vi "Finish.vi"   [LabVIEW 2014]
doc: "This VI is called just before exiting. It is expected to close I/O refnum, save collected data, etc."
uses:
  <vilib>/Rock Robotics/WPI/Joystick/WPI_JoystickGetSetRefNum.vi
  <vilib>/Rock Robotics/WPI/RobotDrive/WPI_RobotDriveGetSetRefNum.vi
  <vilib>/Rock Robotics/WPI/Compressor/WPI_CompressorGetSetRefNum.vi
types:
  T1 = typedef "WPI_JoystickDevRef.ctl" = cluster{"Device":T2}
  T2 = typedef "WPI_JoystickDeviceEnum.ctl" = enum16{"USB 0", "USB 1", "USB 2", "USB 3", "USB 4", "USB 5"}
  T3 = typedef "WPI_RobotDriveDevRef.ctl" = cluster{"DevStatus":errorcluster, "Motors[]":T4[], "Square Inputs":bool, "Max Output":dbl}
  T4 = typedef "WPI_MotorControlDeviceRef.ctl" = cluster{"DeviceStatus":errorcluster, "Type":T5, "PWM":cluster{"Controller":T6, "PWM Channel":T7, "DeadBand":T8}, "CAN":cluster{"Device Number":u8, "Control Mode":T9, "Semaphore":T10, "Max Vout":dbl, "TalonSRX Control Mode":T11}, "Invert":bool, "TransformRef":T12, "InvTransformRef":T12}
  T5 = typedef "WPI_MotorControlType.ctl" = enum16{"PWM", "CAN", "CANTalonSRX"}
  T6 = typedef "FPGA_TypedefDigitalModule.ctl" = enum16{"Controller 1"}
  T7 = typedef "FPGA_DIOPWMChannel.ctl" = enum8{"PWM 0", "PWM 1", "PWM 2", "PWM 3", "PWM 4", "PWM 5", "PWM 6", "PWM 7", "PWM 8", "PWM 9", "PWM MXP 0", "PWM MXP 1", "PWM MXP 2", "PWM MXP 3", "PWM MXP 4", "PWM MXP 5", "PWM MXP 6", "PWM MXP 7", "PWM MXP 8", "PWM MXP 9", "Invalid"}
  T8 = typedef "WPI_PWMDeadband.ctl" = cluster{"Name":string, "maxPositivePwm":i32, "minPositivePwm":i32, "centerPwm":i32, "maxNegativePwm":i32, "minNegativePwm":i32, "angularRange":u16}
  T9 = typedef "WPI_CANJaguar_ControlMode.ctl" = enum8{"Percent VBus", "Current", "Speed", "Position", "Voltage"}
  T10 = typedef "Semaphore RefNum" = refnum<k1>
  T11 = typedef "WPI_CANTalonSRX_APIControlMode.ctl" = enum8{"Percent VBus", "Speed", "Position", "Slave", "Unchanged / Invalid"}
  T12 = typedef "WPI_PWMTransform_ConPane.ctl" = refnum<vi>
  T13 = typedef "WPI_ServoDeviceRef.ctl" = cluster{"DeviceStatus":errorcluster, "Controller":T6, "PWM Channel":T7, "DeadBand":T8}
  T14 = typedef "WPI_DigitalInputDevRef.ctl" = cluster{"DevStatus":errorcluster, "DIO Channel":T15, "Controller":T6}
  T15 = typedef "FPGA_DIOChannel.ctl" = enum8{"DIO 0", "DIO 1", "DIO 2", "DIO 3", "DIO 4", "DIO 5", "DIO 6", "DIO 7", "DIO 8", "DIO 9", "DIO MXP 0", "DIO MXP 1", "DIO MXP 2", "DIO MXP 3", "DIO MXP 4", "DIO MXP 5", "DIO MXP 6", "DIO MXP 7", "DIO MXP 8", "DIO MXP 9", "DIO MXP 10", "DIO MXP 11", "DIO MXP 12", "DIO MXP 13", "DIO MXP 14", "DIO MXP 15", "Invalid"}
  T16 = typedef "WPI_CompressorDevRef.ctl" = cluster{"DevStatus":errorcluster, "Pneumatics Control Module":u8}
  T17 = typedef "WPI_SolenoidDevRef.ctl" = cluster{"DevStatus":errorcluster, "Pneumatics Control Module":u8, "Forward Solenoid Channel":T18, "Reverse Solenoid Channel":T18}
  T18 = typedef "WPI_SolenoidChannel.ctl" = enum8{"Solenoid 0", "Solenoid 1", "Solenoid 2", "Solenoid 3", "Solenoid 4", "Solenoid 5", "Solenoid 6", "Solenoid 7", "Invalid"}
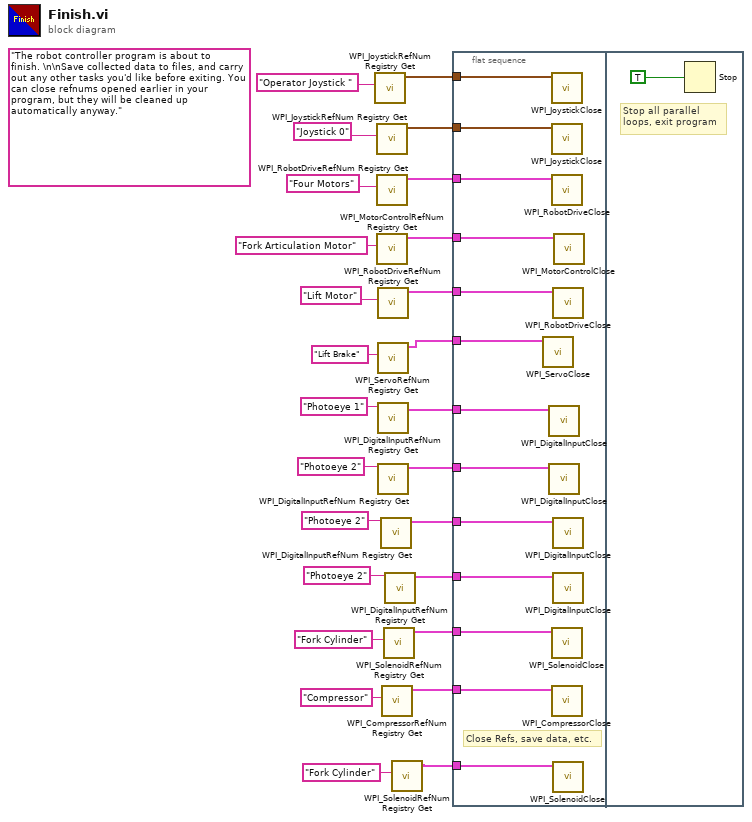
[diagram p0: block diagram]
diagram:
  (unwired) "The robot controller program is about to finish. \n\nSave collected data to files, and carry out any other tasks you'd like before exiting. You can close refnums opened earlier in your program, but they will be cleaned up automatically anyway."
  n1 = call <vilib>:"WPI_JoystickRefNum Registry Get.vi"("refnum name"="Operator Joystick ") -> ("JoystickDevRef"=w21:T1)  [unwired: 9 in, 1 out]
  n2 = call <vilib>:"WPI_JoystickRefNum Registry Get.vi"("refnum name"="Joystick 0") -> ("JoystickDevRef"=w23:T1)  [unwired: 1 in, 9 out]
  n3 = call <vilib>:"WPI_RobotDriveRefNum Registry Get.vi"("refnum name"="Four Motors") -> ("RobotDriveDevRef"=w24:T3)  [unwired: 1 in, 9 out]
  n4 = call <vilib>:"WPI_MotorControlRefNum Registry Get.vi"("refnum name"="Fork Articulation Motor") -> ("MotorControlDevRef"=w19:T4)  [unwired: 9 in, 1 out]
  n5 = call <vilib>:"WPI_RobotDriveRefNum Registry Get.vi"("refnum name"="Lift Motor") -> ("RobotDriveDevRef"=w17:T3)  [unwired: 1 in, 9 out]
  n6 = call <vilib>:"WPI_ServoRefNum Registry Get.vi"("refnum name"="Lift Brake") -> ("ServoDeviceRef"=w6:T13)  [unwired: 9 in, 1 out]
  n7 = call <vilib>:"WPI_DigitalInputRefNum Registry Get.vi"("refnum name"="Photoeye 1") -> ("DigitalInputDevRef"=w11:T14)  [unwired: 9 in, 1 out]
  n8 = call <vilib>:"WPI_DigitalInputRefNum Registry Get.vi"("refnum name"="Photoeye 2") -> ("DigitalInputDevRef"=w9:T14)  [unwired: 9 in, 1 out]
  n9 = call <vilib>:"WPI_DigitalInputRefNum Registry Get.vi"("refnum name"="Photoeye 2") -> ("DigitalInputDevRef"=w10:T14)  [unwired: 9 in, 1 out]
  n10 = call <vilib>:"WPI_CompressorRefNum Registry Get.vi"("refnum name"="Compressor") -> ("CompressorDevRef"=w3:T16)  [unwired: 9 in, 1 out]
  n11 = call <vilib>:"WPI_SolenoidRefNum Registry Get.vi"("refnum name"="Fork Cylinder") -> ("SolenoidDevRef"=w7:T17)  [unwired: 9 in, 1 out]
  n12 = call <vilib>:"WPI_DigitalInputRefNum Registry Get.vi"("refnum name"="Photoeye 2") -> ("DigitalInputDevRef"=w8:T14)  [unwired: 9 in, 1 out]
  n13 = call <vilib>:"WPI_SolenoidRefNum Registry Get.vi"("refnum name"="Fork Cylinder") -> ("SolenoidDevRef"=w1:T17)  [unwired: 9 in, 1 out]
  n14 = flat-sequence {
    tunnel: w24 -> [w39]
    tunnel: w23 -> [w38]
    tunnel: w21 -> [w37]
    tunnel: w19 -> [w36]
    tunnel: w17 -> [w35]
    tunnel: w11 -> [w34]
    tunnel: w10 -> [w33]
    tunnel: w9 -> [w32]
    tunnel: w8 -> [w31]
    tunnel: w7 -> [w30]
    tunnel: w6 -> [w29]
    tunnel: w3 -> [w28]
    tunnel: w1 -> [w27]
    frame #0 {
      # "Close Refs, save data, etc."
      n15 = call <vilib>:"WPI_ServoClose.vi"("ServoDeviceRef"=w29) -> ()  [unwired: 10 in, 1 out]
      n16 = call <vilib>:"WPI_DigitalInputClose.vi"("DigitalInputDevRef"=w34) -> ()  [unwired: 10 in, 1 out]
      n17 = call <vilib>:"WPI_DigitalInputClose.vi"("DigitalInputDevRef"=w32) -> ()  [unwired: 10 in, 1 out]
      n18 = call <vilib>:"WPI_JoystickClose.vi"("JoystickDevRef"=w37) -> ()  [unwired: 11 out]
      n19 = call <vilib>:"WPI_JoystickClose.vi"("JoystickDevRef"=w38) -> ()  [unwired: 11 out]
      n20 = call <vilib>:"WPI_RobotDriveClose.vi"("RobotDriveDevRef"=w39) -> ()  [unwired: 1 in, 10 out]
      n21 = call <vilib>:"WPI_SolenoidClose.vi"("SolenoidDevRef"=w30) -> ()  [unwired: 10 in, 1 out]
      n22 = call <vilib>:"WPI_CompressorClose.vi"("CompressorDevRef"=w28) -> ()  [unwired: 10 in, 1 out]
      n23 = call <vilib>:"WPI_RobotDriveClose.vi"("RobotDriveDevRef"=w35) -> ()  [unwired: 1 in, 10 out]
      n24 = call <vilib>:"WPI_DigitalInputClose.vi"("DigitalInputDevRef"=w33) -> ()  [unwired: 10 in, 1 out]
      n25 = call <vilib>:"WPI_DigitalInputClose.vi"("DigitalInputDevRef"=w31) -> ()  [unwired: 10 in, 1 out]
      n26 = call <vilib>:"WPI_SolenoidClose.vi"("SolenoidDevRef"=w27) -> ()  [unwired: 10 in, 1 out]
      n27 = call <vilib>:"WPI_MotorControlClose.vi"("MotorControlDevRef"=w36) -> ()  [unwired: 10 in, 1 out]
    }
    frame #1 {
      # "Stop all parallel\nloops, exit program"
      n28 = Stop(stop? (T)=TRUE ("Quit")) -> ()
    }
  }
